vi "enable.vi"(8 "error in (no error)":errorcluster, 10 "CommandID":i32, 11 "IContextThisComponent in":refnum<class "IContextThisComponent.lvclass">) -> (0 "error out":errorcluster, 3 "IContextThisComponent out":refnum<class "IContextThisComponent.lvclass">)   [LabVIEW 2016, in "IContextThisComponent.lvclass"]
uses:
  IContextThisComponent.lvclass
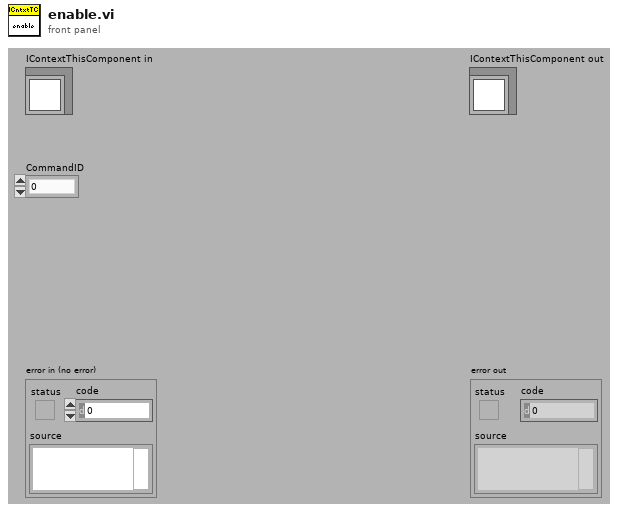
[diagram p1: front panel]
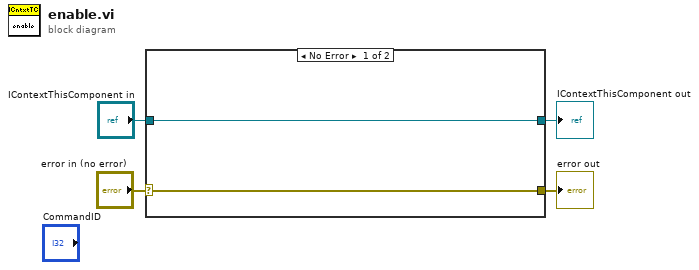
[diagram p0: block diagram]
diagram:
  n1 = case shown="No Error" "error in (no error)" {
    selector: "error in (no error)" -> [w6 w8]
    tunnel: [w6 w8] -> w3
    tunnel: [w5 w7] -> w1
    tunnel: "IContextThisComponent in" -> [w5 w7]
    frame No Error {
    }
    frame Error {
    }
  }
  "error out" <- w3
  "IContextThisComponent out" <- w1
